vi "PutText_TCL.vi"(1 "FlowControlIn":i32, 2 "Node Path":string, 3 "ValueIn":string) -> (0 "FlowControlOut":i32)   [LabVIEW 2011]
panel:
  out "Status":i32
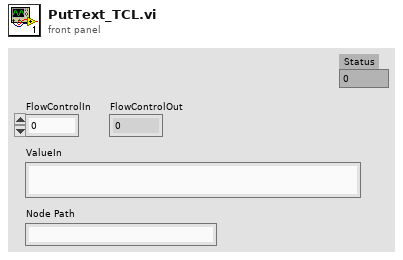
[diagram p1: front panel]
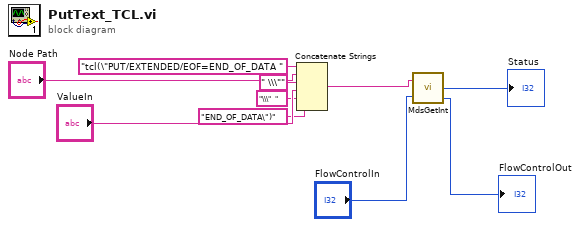
[diagram p0: block diagram]
diagram:
  n1 = Concatenate Strings("tcl(\"PUT/EXTENDED/EOF=END_OF_DATA " ("string"), "Node Path", " \\\"" ("string"), "ValueIn", "\\\"  " ("string"), "END_OF_DATA\")" ("string")) -> (w4:string)
  n2 = call "MdsGetInt.vi"("Expression"=w4, "FlowControlIn"="FlowControlIn") -> ("Status"=→"Status":i32, "FlowControlOut"=→"FlowControlOut":i32)  [unwired: 1 out]
